vi "to_json.vi"(8 "error in":errorcluster, 11 "properties in":refnum<class "properties.lvclass">) -> (0 "error out":errorcluster, 2 "json":string, 3 "properties out":refnum<class "properties.lvclass">)   [LabVIEW 2020, in "nominal types.lvlib" / "properties.lvclass"]
uses:
  properties.lvclass
  properties.lvclass/properties.ctl
  <vilib>/JDP Science/JSONtext/JSONtext.lvlib
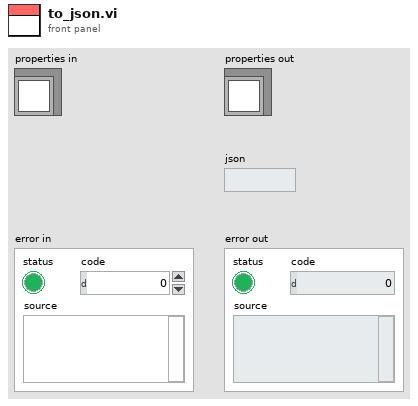
[diagram p1: front panel]
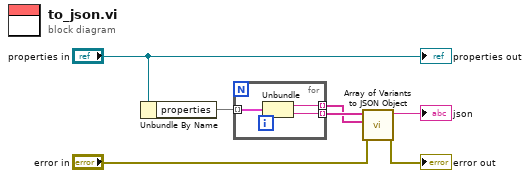
[diagram p0: block diagram]
diagram:
  n1 = Unbundle By Name("properties in") -> ("properties"=w6:map{string, string})
  n2 = for {
    tunnel: w6 -> [w10] mode=indexing
    tunnel: [w9] -> w4 mode=indexing
    tunnel: [w8] -> w5 mode=indexing
    n3 = Unbundle(w10) -> ("name"=w9:string, "value"=w8:string)
  }
  n4 = call <vilib>:"Array of Variants to JSON Object.vi"("error in (no error)"="error in", "Names"=w4, "Array"=w5) -> ("error out"=→"error out":errorcluster, "<JSON>"=→"json":string)  [unwired: 7 in]
  "properties out" <- "properties in"
